vi "Apply.vi"(8 "error in (no error)":errorcluster, 11 "Thermometer DAQmx Base CFG in":refnum<class "Thermometer DAQmx Base CFG.lvclass">) -> (0 "error out":errorcluster, 3 "Thermometer DAQmx Base CFG out":refnum<class "Thermometer DAQmx Base CFG.lvclass">)   [LabVIEW 2023, in "Thermometer DAQmx Base CFG.lvlib" / "Thermometer DAQmx Base CFG.lvclass"]
uses:
  Thermometer DAQmx Base CFG.lvclass
  Thermometer DAQmx Base CFG.lvclass/Thermometer DAQmx Base CFG.ctl
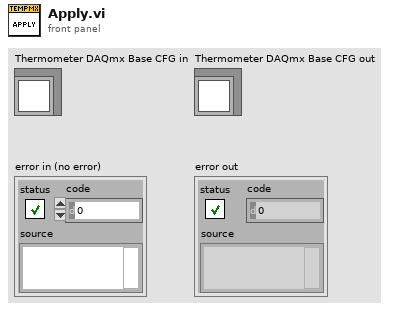
[diagram p1: front panel]
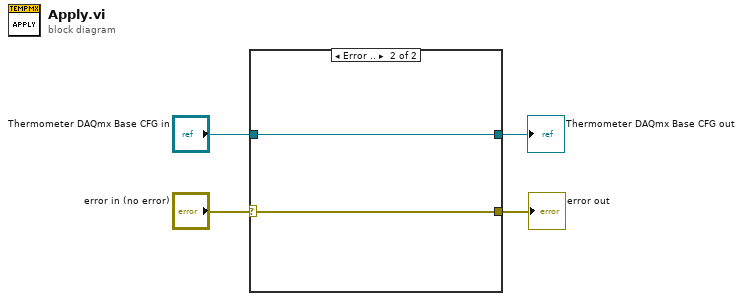
[diagram p0: block diagram]
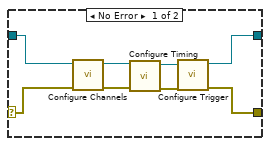
[diagram p2: hidden frame]
diagram:
  n1 = case shown="Error .." "error in (no error)" {
    selector: "error in (no error)" -> [w5 w13]
    tunnel: "Thermometer DAQmx Base CFG in" -> [w6 w14]
    tunnel: [w8 w13] -> w2
    tunnel: [w7 w14] -> w1
    frame No Error {
      n2 = call-dynamic "Configure Channels.vi"("error in (no error)"=w5, "Thermometer DAQmx Base CFG in"=w6) -> ("error out"=w11:errorcluster, "Thermometer DAQmx Base CFG out"=w12:refnum<class "Thermometer DAQmx Base CFG.lvclass">)  [unwired: 8 in]
      n3 = call-dynamic "Configure Timing.vi"("error in (no error)"=w11, "Thermometer DAQmx Base CFG in"=w12) -> ("error out"=w9:errorcluster, "Thermometer DAQmx Base CFG out"=w10:refnum<class "Thermometer DAQmx Base CFG.lvclass">)  [unwired: 8 in]
      n4 = call-dynamic "Configure Trigger.vi"("error in (no error)"=w9, "Thermometer DAQmx Base CFG in"=w10) -> ("error out"=w8:errorcluster, "Thermometer DAQmx Base CFG out"=w7:refnum<class "Thermometer DAQmx Base CFG.lvclass">)  [unwired: 8 in]
    }
    frame Error {
    }
  }
  "error out" <- w2
  "Thermometer DAQmx Base CFG out" <- w1
